vi "PotenciometroError.vi"(8 "error in (no error)":errorcluster, 9 "Wavelength (0.0)":dbl, 11 "num Lect":i32) -> (0 "error out":errorcluster, 2 "Valor Prom":dbl)   [LabVIEW 2018]
uses:
  <vilib>/Utility/error.llb/DialogType.ctl
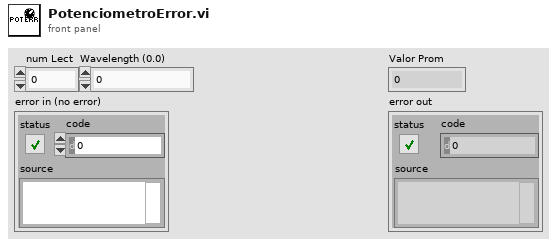
[diagram p1: front panel]
types:
  T1 = typedef "DialogType.ctl" = u16
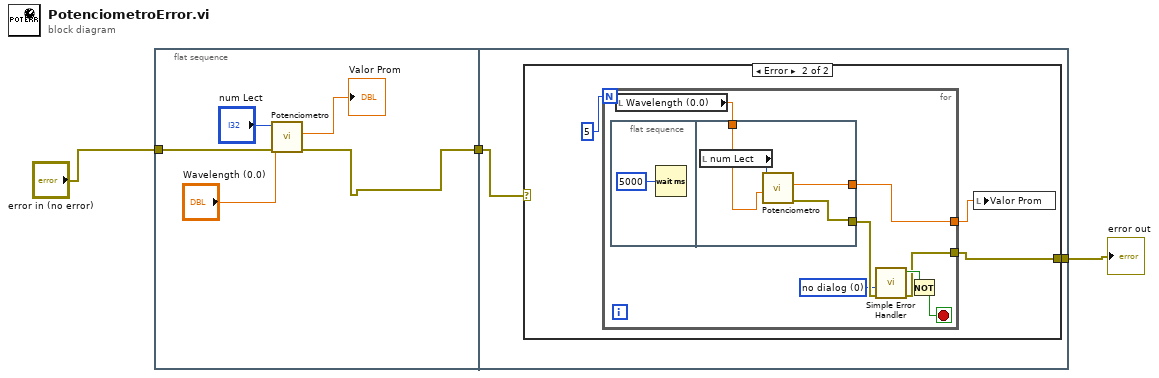
[diagram p0: block diagram]
diagram:
  n1 = flat-sequence {
    tunnel: [w6] -> w3
    tunnel: "error in (no error)" -> [w5]
    tunnel: w3 -> [w10]
    tunnel: [w9] -> w2
    frame #0 {
      n2 = call "Potenciometro.vi"("error in (no error)"=w5, "Wavelength (0.0)"="Wavelength (0.0)", "num Lect"="num Lect") -> ("error out"=w6:errorcluster, "Valor Prom"=→"Valor Prom":dbl)  [unwired: 6 in, 1 out]
    }
    frame #1 {
      n3 = case shown="Error" w10 {
        selector: w10 -> [w11 _]
        tunnel: [w11 w12] -> w9
        frame No Error {
        }
        frame Error {
          n4 = for {
            N: 5 -> [_]
            tunnel: [w21] -> w13
            tunnel: [w17] -> w12
            stop <- w18 stop-if-true
            w16 = T1 0 items=["no dialog", "OK message", "continue or stop message", "OK message + warnings", "continue/stop + warnings"] ("type of dialog (OK msg:1)")
            n5 = flat-sequence {
              tunnel: [w25] -> w21
              tunnel: [w24] -> w20
              tunnel: w15 -> [w23]
              frame #0 {
                n6 = Wait (ms)(milliseconds to wait=u32 5000) -> ()  [unwired: 1 out]
              }
              frame #1 {
                n7 = local read "num Lect"() -> (w26:i32)
                n8 = call "Potenciometro.vi"("Wavelength (0.0)"=w23, "num Lect"=w26) -> ("error out"=w24:errorcluster, "Valor Prom"=w25:dbl)  [unwired: 7 in, 1 out]
              }
            }
            n9 = local read "Wavelength (0.0)"() -> (w15:dbl)
            n10 = call <vilib>:"Simple Error Handler.vi"("type of dialog (OK msg:1)"=w16, "error in (no error)"=w20) -> ("error?"=w19:bool, "error out"=w17:errorcluster)  [unwired: 3 in, 3 out]
            n11 = Not(x=w19) -> (.not. x?=w18:bool)
          }
          n12 = local write "Valor Prom"(w13) -> ()
        }
      }
    }
  }
  "error out" <- w2
